vi "Search and Replace Multiple Patterns.vi"(7 "replace all? (F)":bool, 8 "offset (0)":i32, 9 "replace strings (\"\")":string[](array[string]), 10 "regular expressions":string[](array[string]), 11 "source":string) -> (1 "offsets past match":i32[](array[numeric]), 3 "result string":string)   [LabVIEW 2021]
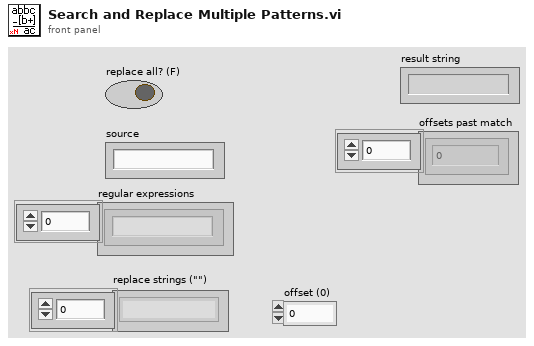
[diagram p1: front panel]
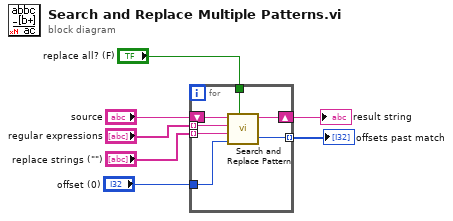
[diagram p0: block diagram]
diagram:
  n1 = for {
    tunnel: "regular expressions" -> [w14] mode=indexing
    tunnel: "replace all? (F)" -> [w13]
    tunnel: "replace strings (\"\")" -> [w10] mode=indexing
    shift-right: [w11] -> w4
    shift-left: "source" -> [w12]
    tunnel: "offset (0)" -> [w9]
    tunnel: [w8] -> w1 mode=indexing
    n2 = call <vilib>:"Search and Replace Pattern.vi"("string"=w12, "regular expression (\"\")"=w14, "replace string (\"\")"=w10, "offset (0)"=w9, "replace all? (F)"=w13) -> ("result string"=w11:string, "offset past match"=w8:i32)
  }
  "result string" <- w4
  "offsets past match" <- w1
